vi "Global - Device Input.vi"() -> ()   [LabVIEW 2019]
panel:
  in  "Device Input":string[](array[string])
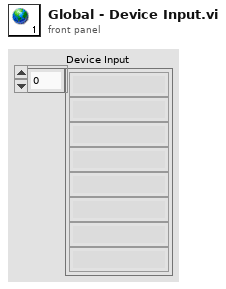
[diagram p1: front panel]
diagram:
